vi "Create.vi"(7 "Size (32x32)":cluster{"Width":u16, "Height":u16}={"Width"=32, "Height"=32}, 8 "error in (no error)":errorcluster, 10 "Index (42)":i32=42, 11 "Tree":refnum<vi>) -> (0 "error out":errorcluster, 3 "Picture Control Canvas out":refnum<class "Tree Control Canvas.lvclass">)   [LabVIEW 2023, in "Font Glyph Drawer Interface.lvlib" / "Tree Control Canvas.lvclass"]
uses:
  Tree Control Canvas.lvclass
  Tree Control Canvas.lvclass/Tree Control Canvas.ctl
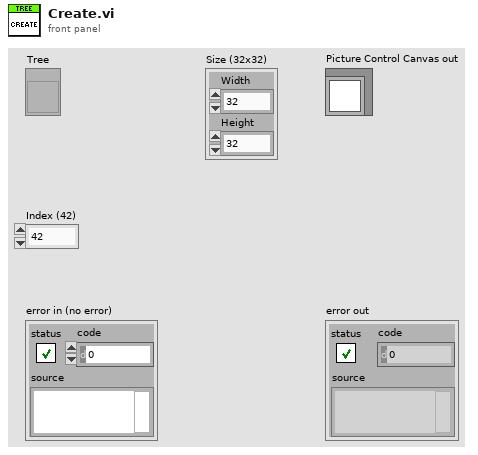
[diagram p1: front panel]
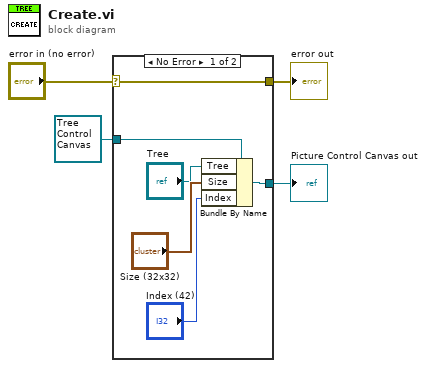
[diagram p0: block diagram]
diagram:
  n1 = case shown="No Error" "error in (no error)" {
    selector: "error in (no error)" -> [w9 w12]
    tunnel: [w9 w12] -> w3
    tunnel: [w8 w11] -> w1
    tunnel: refnum<class "Tree Control Canvas.lvclass"> refnum ("Picture Control Canvas in") -> [w10 w11]
    frame No Error {
      n2 = Bundle By Name(cluster=w10, "Tree"="Tree", "Size"="Size (32x32)", "Index"="Index (42)") -> (w8:refnum<class "Tree Control Canvas.lvclass">)
    }
    frame Error {
    }
  }
  "error out" <- w3
  "Picture Control Canvas out" <- w1
